vi "Target.vi"() -> ()   [LabVIEW 2018]
uses:
  <vilib>/Platform/TimedLoop/XDataNode/timing_clust.ctl
  <vilib>/Platform/TimedLoop/XDataNode/nitl_modes.ctl
  <vilib>/Platform/TimedLoop/XDataNode/wakeup.ctl
  <vilib>/rvi/eio/common/nirviEmuTemplateMethod_errors.vi
  <vilib>/rvi/Emulation/niFpgaSctlEmulationGetInTimedLoop.vi
  <vilib>/rvi/Emulation/niFpgaEmulationReportErrorSimple.vi
  <vilib>/rvi/Emulation/niFpgaGetClockAttributes.vi
  <vilib>/rvi/Emulation/niFpgaCriticalErrorInLSC.vi
  <vilib>/rvi/Emulation/niFpgaProcessEmulError.vi
  <vilib>/eio/EIONode/EIONode.xnode
  <vilib>/Platform/TimedLoop/XDataNode/XDataNode.xnode
  <vilib>/Platform/TimedLoop/XDataNode/XDNodeRunTimeDep.lvlib
panel:
  in  "RESET":bool=TRUE
  in  "30":i32=30
  in  "20":i32=20
  in  "40":i32=40
  in  "A0":bool
  in  "10":i32=10
  in  "DATA":u8
  in  "Stop_FPGA":bool
  in  "Запись":bool
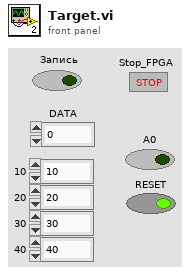
[diagram p1: front panel]
types:
  T1 = typedef "XDNodeRunTimeDep.lvlib/timing_clust.ctl" = cluster{"Expected End [f-1]":u64, "Actual End [f-1]":u64, "Finished Late? [f-1]":bool, "Expected End [i-1]":u64, "Actual End [i-1]":u64, "Finished Late? [i-1]":bool, "Expected Start [i]":u64, "Actual Start [i]":u64, "Expected Start [f]":u64, "Actual Start [f]":u64, "Source Name":string, "Structure Name":string, "Period":i64, "Deadline":i64, "Offset":i64, "Start":i64, "Priority":i32, "Timeout":i32, "Mode":T2, "Wakeup Reason":T3, "Error":errorcluster, "Source Type":string, "Secondary Source Type":string, "Global End Time":u64, "Global Start Time":u64, "Frame Duration":u64, "Iteration Duration":u64, "Assigned CPU":i32, "I/O Scan Engine Mode":u32}
  T2 = typedef "XDNodeRunTimeDep.lvlib/nitl_modes.ctl" = enum32{"No Change", "Process missed periods, maintain original phase", "Discard missed periods, maintain original phase", "Process missed periods, ignore original phase", "Discard missed periods, ignore original phase"}
  T3 = typedef "XDNodeRunTimeDep.lvlib/wakeup.ctl" = enum32{"Normal", "Aborted", "Asynchronous wakeup", "Timing source error", "Timed loop error", "Timeout"}
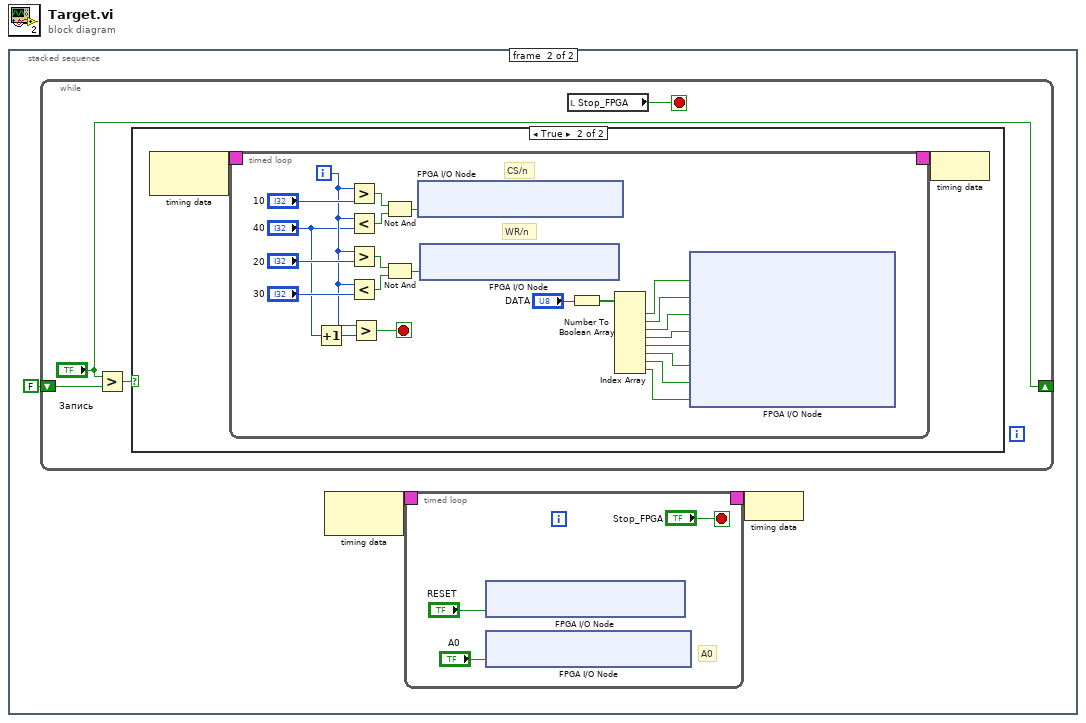
[diagram p0: block diagram]
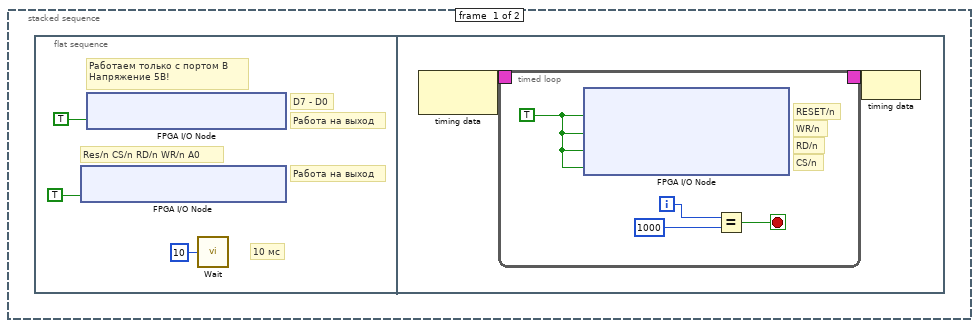
[diagram p2: hidden frame]
diagram:
  n1 = stacked-sequence {
    frame #0 {
      n2 = flat-sequence {
        frame #0 {
          # "Res/n CS/n RD/n WR/n A0"
          # "D7 - D0"
          # "Работа на выход"
          # "10 мс"
          # "Работа на выход"
          # "Работаем только с портом B\nНапряжение 5В!"
          n3 = xnode "FPGA I/O Node"("IO Module\\DDCB_DIO8-15_WE"=TRUE ("IO Module\\DDCA_DIO8-15_WE")) -> ()  [unwired: 1 in, 1 out]
          n4 = xnode "FPGA I/O Node"("IO Module\\DDCB_DIO0-7_WE"=TRUE ("IO Module\\DDCA_DIO0-7_WE")) -> ()  [unwired: 1 in, 1 out]
          n5 = call "Wait"("Count(mSec)"=u8 10 ("Count(uSec)")) -> ()  [unwired: 1 out]
        }
        frame #1 {
          n6 = node-c288() -> (w5:T1)  [unwired: 1 in]
          n7 = timed-loop {
            timing: w5 -> [_]
            timing-out: [_] -> w4
            i -> [w8]
            stop <- w9 stop-if-true
            w6 = TRUE ("IO Module\\DDCB_DIO8_Write")
            # "CS/n"
            # "RD/n"
            # "WR/n"
            # "RESET/n"
            n8 = xnode "FPGA I/O Node"("IO Module\\DDCB_DIO8_Write"=w6, "IO Module\\DDCB_DIO9_Write"=w6, "IO Module\\DDCB_DIO10_Write"=w6, "IO Module\\DDCB_DIO11_Write"=w6) -> ()  [unwired: 4 in, 4 out]
            n9 = Equal?(x=w8, y=1000) -> (x = y?=w9:bool)
          }
          n10 = node-c288(w4) -> ()
        }
      }
    }
    frame #1 {
      n11 = while {
        shift-right: ["Запись"] -> _
        shift-left: FALSE ("SPI") -> [w26]
        stop <- w24 stop-if-true
        n12 = Greater?(x="Запись", y=w26) -> (0:w27:bool)
        n13 = case shown="True" w27 {
          frame False {
          }
          frame True {
            n14 = node-c288() -> (w29:T1)  [unwired: 1 in]
            n15 = timed-loop {
              timing: w29 -> [_]
              timing-out: [_] -> w28
              i -> [w40]
              stop <- w30 stop-if-true
              # "CS/n"
              # "WR/n"
              n16 = Increment(x="40") -> (x+1=w32:i32)
              n17 = Greater?(x=w40, y="10") -> (0:w48:bool)
              n18 = Less?(x=w40, y="40") -> (x < y?=w47:bool)
              n19 = Greater?(x=w40, y="20") -> (0:w44:bool)
              n20 = Less?(x=w40, y="30") -> (x < y?=w43:bool)
              n21 = Greater?(x=w40, y=w32) -> (0:w30:bool)
              n22 = Not And(1:w47, 2:w48) -> (0:w42:bool)
              n23 = Not And(1:w43, 2:w44) -> (0:w41:bool)
              n24 = xnode "FPGA I/O Node"("IO Module\\DDCB_DIO11_Write"=w42) -> ()  [unwired: 1 in, 1 out]
              n25 = xnode "FPGA I/O Node"("IO Module\\DDCB_DIO9_Write"=w41) -> ()  [unwired: 1 in, 1 out]
              n26 = Number To Boolean Array(number="DATA") -> (Boolean array=w51:bool[])
              n27 = Index Array(array=w51) -> (element #1=w50:bool, element #2=w39:bool, element #3=w38:bool, element #4=w37:bool, element #5=w36:bool, element #6=w35:bool, element #7=w34:bool, element #8=w33:bool)  [unwired: 8 in]
              n28 = xnode "FPGA I/O Node"("IO Module\\DDCB_DIO0_Write"=w50, "IO Module\\DDCB_DIO1_Write"=w39, "IO Module\\DDCB_DIO13_Write"=w38, "IO Module\\DDCB_DIO3_Write"=w37, "IO Module\\DDCB_DIO4_Write"=w36, "IO Module\\DDCB_DIO5_Write"=w35, "IO Module\\DDCB_DIO6_Write"=w34, "IO Module\\DDCB_DIO7_Write"=w33) -> ()  [unwired: 8 in, 8 out]
            }
            n29 = node-c288(w28) -> ()
          }
        }
        n30 = local read "Stop_FPGA"() -> (w24:bool)
      }
      n31 = node-c288() -> (w15:T1)  [unwired: 1 in]
      n32 = timed-loop {
        timing: w15 -> [_]
        timing-out: [_] -> w14
        stop <- "Stop_FPGA" stop-if-true
        # "A0"
        n33 = xnode "FPGA I/O Node"("IO Module\\DDCB_DIO8_Write"="RESET") -> ()  [unwired: 1 in, 1 out]
        n34 = xnode "FPGA I/O Node"("IO Module\\DDCB_DIO12_Write"="A0") -> ()  [unwired: 1 in, 1 out]
      }
      n35 = node-c288(w14) -> ()
    }
  }
